vi "GetMeasurementMatrix.vi"(7 "error in":errorcluster, 9 "lsecon":T2={"NoiseVariance"=0.001, "IEEESystem"=5, "PMULocations"=[1], "Vindex"=0, "Iindex"=3, "DynamicRef"=""}, 10 "PMUnumber":i32=1) -> (0 "error out":errorcluster, 2 "SystemVoltagesRef":cdb[][](array[numeric]), 3 "NetworkData":T1)   [LabVIEW 2014, in "AppPlugins.lvlib" / "LSEPlugin.lvclass"]
uses:
  LSEPlugin.lvclass
  Typedefs/LSEConfig.ctl
  Typedefs/Network.ctl
panel:
  out "2-D Array of Real":dbl[][](array[numeric])
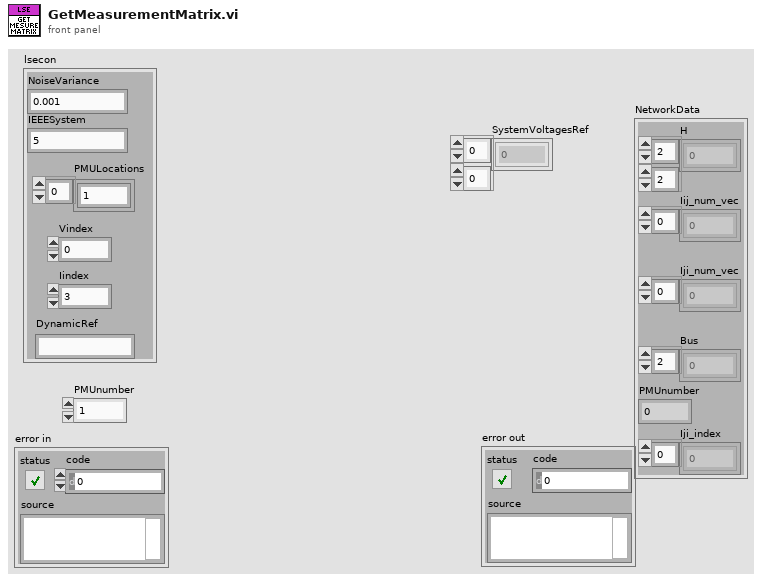
[diagram p1: front panel]
types:
  T1 = typedef "AppPlugins.lvlib/LSEPlugin.lvclass/Network.ctl" = cluster{"H":dbl[][], "Iij_num_vec":dbl[], "Iji_num_vec":dbl[], "Bus":dbl[], "PMUnumber":i32, "Iji_index":i32[]}
  T2 = typedef "AppPlugins.lvlib/LSEPlugin.lvclass/LSEConfig.ctl" = cluster{"NoiseVariance":dbl, "IEEESystem":u32, "PMULocations":u32[], "Vindex":i32, "Iindex":i32, "DynamicRef":string}
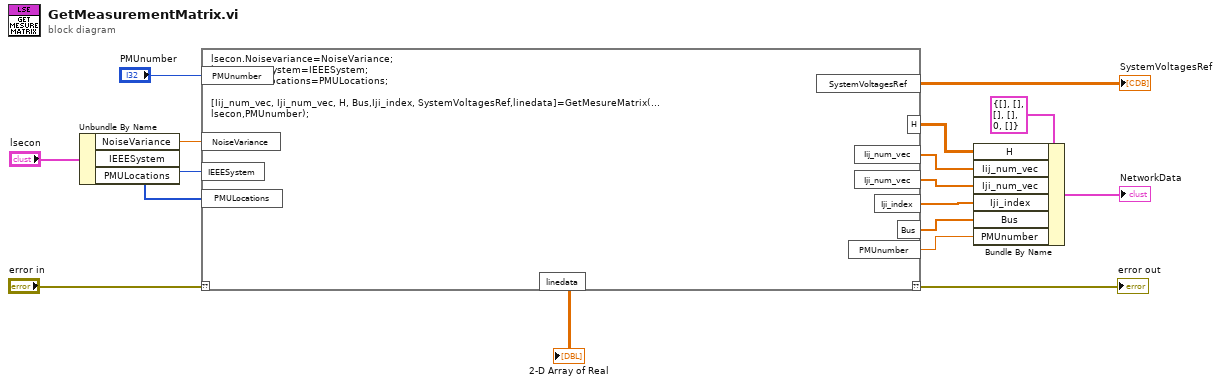
[diagram p0: block diagram]
diagram:
  n1 = Unbundle By Name("lsecon") -> ("NoiseVariance"=w14:dbl, "IEEESystem"=w13:u32, "PMULocations"=w12:u32[])
  n2 = script code="lsecon.Noisevariance=NoiseVariance; \nlsecon.IEEESystem=IEEESystem;\nlsecon.PMULocations=PMULocations;\n\n[Iij_num_vec, Iji_num_vec, H, Bus,Iji_index, SystemVoltagesRef,linedata]=GetMesureMatrix(...\nlsecon,PMUnumber);"("??"="error in", "PMUnumber"="PMUnumber", "NoiseVariance"=w14, "IEEESystem"=w13, "PMULocations"=w12) -> ("??"=→"error out":errorcluster, "SystemVoltagesRef"=→"SystemVoltagesRef":cdb[][], "H"=w10:dbl[][], "Iij_num_vec"=w5:dbl[], "Iji_num_vec"=w9:dbl[], "Bus"=w7:dbl[], "PMUnumber"=w6:dbl, "Iji_index"=w8:dbl[], "linedata"=→"2-D Array of Real":dbl[][])
  n3 = Bundle By Name(cluster=T1 {"H"=[], "Iij_num_vec"=[], "Iji_num_vec"=[], "Bus"=[], "PMUnumber"=0, "Iji_index"=[]} ("network_data"), "H"=w10, "Iij_num_vec"=w5, "Iji_num_vec"=w9, "Iji_index"=w8, "Bus"=w7, "PMUnumber"=w6) -> (→"NetworkData":T1)
